vi "readConfigCmd.vi"(8 "error in (no error)":errorcluster, 11 "Path in":T1) -> (0 "error out":errorcluster, 2 "regCmd":string[](array[string]), 3 "Path out":T1)   [LabVIEW 2018]
doc: "Read commands from default.ini file that will be registered by TCP Server.\n\nNOTE: this is only for internal use. User does not call this function directly."
uses:
  <vilib>/Utility/config.llb/Config Data RefNum.ctl
  <vilib>/Utility/config.llb/NI_LVConfig.lvlib
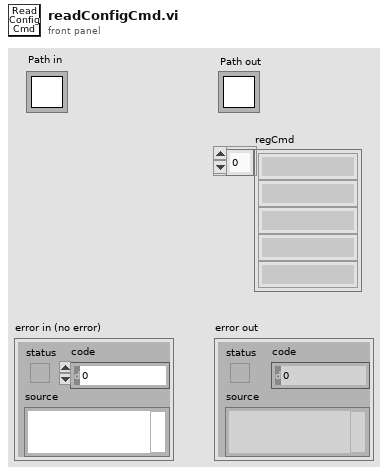
[diagram p1: front panel]
types:
  T1 = typedef "NI_LVConfig.lvlib/Config Data RefNum.ctl" = refnum<k1>
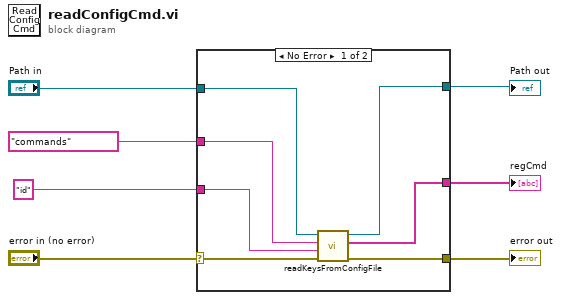
[diagram p0: block diagram]
diagram:
  n1 = case shown="No Error" "error in (no error)" {
    selector: "error in (no error)" -> [w10 w16]
    tunnel: "id" -> [w9 _]
    tunnel: "commands" -> [w14 _]
    tunnel: [w13 w15] -> w2
    tunnel: [w12 _] -> w1
    tunnel: "Path in" -> [w8 w15]
    tunnel: [w11 w16] -> w3
    frame No Error {
      n2 = call "readKeysFromConfigFile.vi"("error in (no error)"=w10, "keys"=w9, "section"=w14, "Refnum in"=w8) -> ("error out"=w11:errorcluster, "arrayOfKeys"=w12:string[], "Refnum out"=w13:T1)  [unwired: 5 in]
    }
    frame Error {
    }
  }
  "regCmd" <- w1
  "error out" <- w3
  "Path out" <- w2
